vi "lua_pcall.vi"(0 "lua_State *L":u64, 5 "nargs":i32, 7 "nresults":i32, 9 "errfunc":i32, 11 "error in":errorcluster) -> (4 "lua_pcall":i32(ring) items=["LUA_OK", "LUA_YIELD", "LUA_ERRRUN", "LUA_ERRSYNTAX", "LUA_ERRMEM", "LUA_ERRERR"], 15 "error out":errorcluster)   [LabVIEW 2011]
doc: "int lua_pcall (lua_State *L, int nargs, int nresults, int errfunc);\nCalls a function in protected mode. \n\nBoth nargs and nresults have the same meaning as in lua_call. If there are no errors during the call, lua_pcall behaves exactly like lua_call. However, if there is any error, lua_pcall catches it, pushes a single value on the stack (the error message), and returns an error code. Like lua_call, lua_pcall always removes the function and its arguments from the stack. \n\nIf errfunc is 0, then the error message returned on the stack is exactly the original error message. Otherwise, errfunc is the stack index of an error handler function. (In the current implementation, this index cannot be a pseudo-index.) In case of runtime errors, this function will be called with the error message and its return value will be the message returned on the stack by lua_pcall. \n\nTypically, the error handler function is used to add more debug information to the error message, such as a stack traceback. Such information cannot be gathered after the return of lua_pcall, since by then the stack has unwound. \n\nThe lua_pcall function returns 0 in case of success or one of the following error codes (defined in lua.h): \nc\nLUA_ERRRUN: a runtime error. \nLUA_ERRMEM: memory allocation error. For such errors, Lua does not call the error handler function. \nLUA_ERRERR: error while running the error handler function."
uses:
  lua5.1.dll
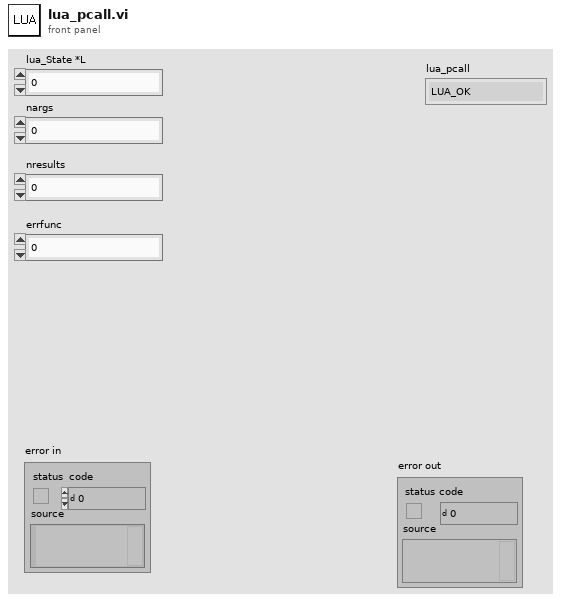
[diagram p1: front panel]
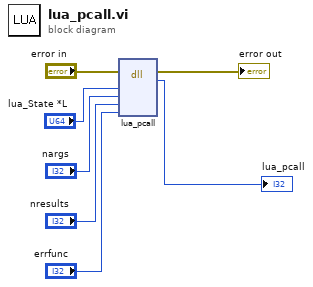
[diagram p0: block diagram]
diagram:
  n1 = dll-call lib="G:/_baidu_backup/monkey task 2012/source program/LuaDllToLabview/lowlevel/lua5.1.dll" fn="lua_pcall"(error in="error in", "lua_State *L"="lua_State *L", "nargs"="nargs", "nresults"="nresults", "errfunc"="errfunc") -> (error out=→"error out":errorcluster, "lua_pcall"=→"lua_pcall":i32)  [unwired: 6 in, 1 out]
